vi "metadata_GetAttributes.vi"(0 "reference in":refnum<class "metadata.lvclass">, 1 "return data? (T)":bool=TRUE, 5 "error in (no error)":errorcluster) -> (14 "reference out":refnum<class "metadata.lvclass">, 15 "attributes ref":T13, 16 "attributes":T1={"MyAttribute"=0.0, "System Control"={"FPGA SW version"="", "TDMS file version"="", "Instrument"="", "Instrument model"="", "Instrument scanner"="", "Instrument clockrate (Mhz)"="", "Instrument tick time (us)"=""}, "file info"={"Time Stamp"=timestamp(0 s since 1904-01-01), "Filename"="", "Filepath"=path "", "User"="", "Experiment_name"="", "Curve_id"="", "number_segments"=0, "number_consecutive_scans"=0}, "Sample info"={"Sample name"="", "Sample species"=""}, "Cantilever info"={"spring constant calib method"="", "invOLS calib method"="", "thermal calib deflection channel"="", "model"="", "shape"="", "tip geometry"="", "Laser sum (V)"=0.0, "Laser power (mA)"=0.0, "invOLS_(nm/V)"=0.0, "spring constant nominal (N/m)"=0.0, "spring constant calib (N/m)"=0.0, "resosnance frequency air calib (Hz)"=0.0, "resosnance frequency calib (Hz)"=0.0, "quality factor"=0.0, "Acoefficident_GCI_(nN.s^1.3/m)"=0.0, "half angle (deg)"=0.0, "tip radius (m)"=0.0, "tip height (m)"=0.0, "system mount angle (deg)"=0.0}, "XYZ piezos"={"X stage piezo sensitivity (nm/V)"=0.0, "X stage piezo gain"=0.0, "X velocity (V/tick)"=0.0, "X closed loop"=FALSE, "Y stage piezo sensitivity (nm/V)"=0.0, "Y stage piezo gain"=0.0, "Y velocity (V/tick)"=0.0, "Y closed loop"=FALSE, "Z stage piezo sensitivity (nm/V)"=0.0, "Z stage piezo gain"=0.0, "Z closed loop"=FALSE, "X position (V)"=0.0, "Y position (V)"=0.0}, "Mapping"={"Mapping"=FALSE, "index"=0, "position row"=0, "position column"=0, "next position row"=0, "next position column"=0, "X initial position (V)"=0.0, "Y initial position (V)"=0.0, "X step size (V)"=0.0, "Y step size (V)"=0.0}, "Fcurve segment"=[], "Fast fpga segment"={"Fast start time trigger"=timestamp(0 s since 1904-01-01), "nb_points"=0, "sampling_rate_(S/s)"=0, "duration_(ticks)"=0}, "Chirp"={"f start (Hz)"=0.0, "f end (Hz)"=0.0, "Sweep type"=""}, "precision (6)"=6, "width (-)"=0, "Metadata"={"Property Names"=[], "Property Values"=[]}, "config filepath"=path "", "Section names []"=[], "Property names []"=[], "nb elements"=0}, 19 "error out":errorcluster)   [LabVIEW 2019, in "metadata.lvclass"]
doc: "Returns a reference and if wanted the actual data values of the attributes. This method is used by the subclasses to access parent attributes."
uses:
  metadata.lvclass
  C:/Program Files/National Instruments/LabVIEW 2019/vi.lib/addons/_AddQ/G#Object/G#Object.lvclass
  ObjectAttributesRef.ctl
  protected/ObjectAttributes.ctl
  System control parameters.ctl
  File info parameters.ctl
  Sample info parameters.ctl
  Cantilever info parameters.ctl
  XYZ piezos parameters.ctl
  Mapping parameters.ctl
  Fcurve segment.ctl
  Segment type--combobox.ctl
  fast fpga segment parameters.ctl
  Chirp added parameters.ctl
  Metadata output --cluster.ctl
  metadata.lvclass/metadata.ctl
  <vilib>/addons/_AddQ/G#Object/G#Object.lvclass
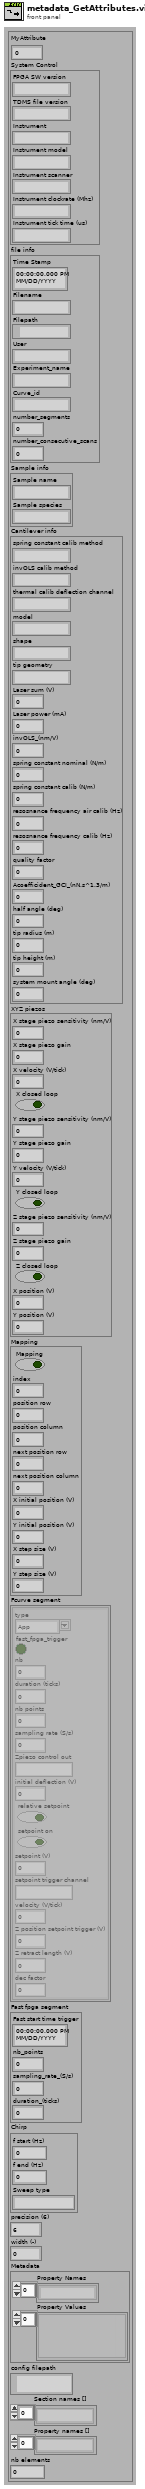
[diagram p1: front panel]
types:
  T1 = typedef "metadata.lvclass/ObjectAttributes.ctl" = cluster{"MyAttribute":dbl, "System Control":T2, "file info":T3, "Sample info":T4, "Cantilever info":T5, "XYZ piezos":T6, "Mapping":T7, "Fcurve segment":T8[], "Fast fpga segment":T10, "Chirp":T11, "precision (6)":i16, "width (-)":i16, "Metadata":T12, "config filepath":path, "Section names []":string[], "Property names []":string[], "nb elements":u16}
  T2 = typedef "metadata.lvclass/System control parameters.ctl" = cluster{"FPGA SW version":string, "TDMS file version":string, "Instrument":string, "Instrument model":string, "Instrument scanner":string, "Instrument clockrate (Mhz)":string, "Instrument tick time (us)":string}
  T3 = typedef "metadata.lvclass/File info parameters.ctl" = cluster{"Time Stamp":timestamp, "Filename":string, "Filepath":path, "User":string, "Experiment_name":string, "Curve_id":string, "number_segments":u8, "number_consecutive_scans":u32}
  T4 = typedef "metadata.lvclass/Sample info parameters.ctl" = cluster{"Sample name":string, "Sample species":string}
  T5 = typedef "metadata.lvclass/Cantilever info parameters.ctl" = cluster{"spring constant calib method":string, "invOLS calib method":string, "thermal calib deflection channel":string, "model":string, "shape":string, "tip geometry":string, "Laser sum (V)":dbl, "Laser power (mA)":dbl, "invOLS_(nm/V)":dbl, "spring constant nominal (N/m)":dbl, "spring constant calib (N/m)":dbl, "resosnance frequency air calib (Hz)":dbl, "resosnance frequency calib (Hz)":dbl, "quality factor":dbl, "Acoefficident_GCI_(nN.s^1.3/m)":dbl, "half angle (deg)":dbl, "tip radius (m)":dbl, "tip height (m)":dbl, "system mount angle (deg)":dbl}
  T6 = typedef "metadata.lvclass/XYZ piezos parameters.ctl" = cluster{"X stage piezo sensitivity (nm/V)":dbl, "X stage piezo gain":dbl, "X velocity (V/tick)":dbl, "X closed loop":bool, "Y stage piezo sensitivity (nm/V)":dbl, "Y stage piezo gain":dbl, "Y velocity (V/tick)":dbl, "Y closed loop":bool, "Z stage piezo sensitivity (nm/V)":dbl, "Z stage piezo gain":dbl, "Z closed loop":bool, "X position (V)":dbl, "Y position (V)":dbl}
  T7 = typedef "metadata.lvclass/Mapping parameters.ctl" = cluster{"Mapping":bool, "index":u16, "position row":u16, "position column":u16, "next position row":i16, "next position column":i16, "X initial position (V)":dbl, "Y initial position (V)":dbl, "X step size (V)":dbl, "Y step size (V)":dbl}
  T8 = typedef "metadata.lvclass/Fcurve segment.ctl" = cluster{"type":T9, "fast_fpga_trigger":bool, "nb":u8, "duration (ticks)":i64, "nb points":i32, "sampling rate (S/s)":u32, "Zpiezo control out":string, "initial deflection (V)":dbl, "relative setpoint":bool, "setpoint on":bool, "setpoint (V)":dbl, "setpoint trigger channel":string, "velocity (V/tick)":dbl, "Z position setpoint trigger (V)":dbl, "Z retract length (V)":dbl, "dec factor":u32}
  T9 = typedef "metadata.lvclass/Segment type--combobox.ctl" = string
  T10 = typedef "metadata.lvclass/fast fpga segment parameters.ctl" = cluster{"Fast start time trigger":timestamp, "nb_points":u32, "sampling_rate_(S/s)":u32, "duration_(ticks)":u32}
  T11 = typedef "metadata.lvclass/Chirp added parameters.ctl" = cluster{"f start (Hz)":dbl, "f end (Hz)":dbl, "Sweep type":string}
  T12 = typedef "metadata.lvclass/Metadata output --cluster.ctl" = cluster{"Property Names":string[], "Property Values":variant[]}
  T13 = typedef "metadata.lvclass/ObjectAttributesRef.ctl" = refnum<data-value>
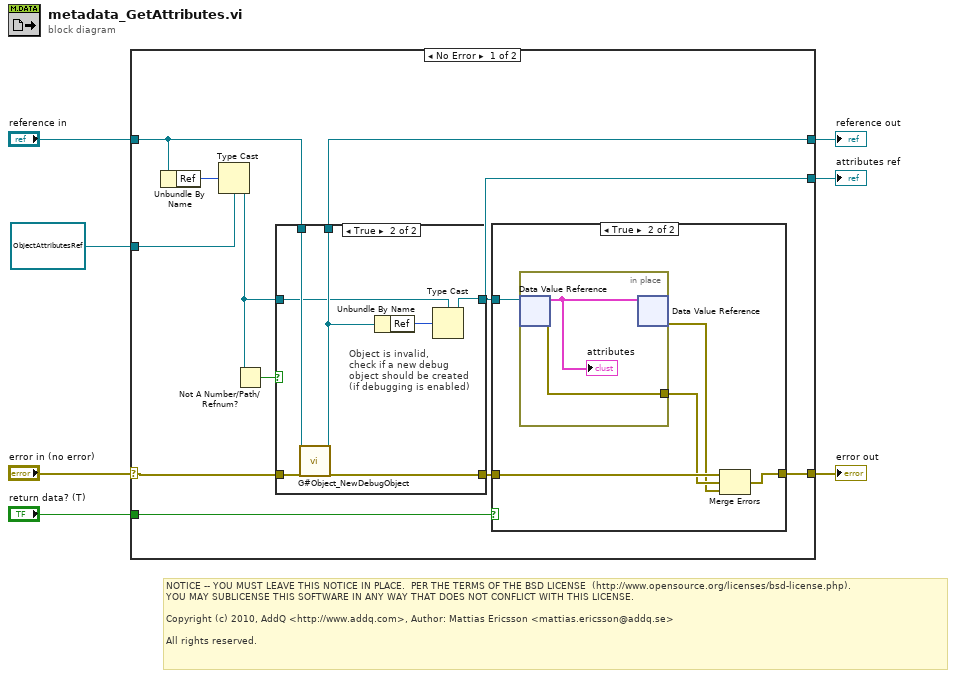
[diagram p0: block diagram]
diagram:
  # "NOTICE -- YOU MUST LEAVE THIS NOTICE IN PLACE.  PER THE TERMS OF THE BSD LICENSE  (http://www.opensource.org/licenses/bsd-license.php).\nYOU MAY SUBLICENSE THIS SOFTWARE IN ANY WAY THAT DOES NOT CONFLICT WITH THIS LICENSE.\n\nCopyright (c) 2010, AddQ <http://www.addq.com>, Author: Mattias Ericsson <mattias.ericsson@addq.se>\n\nAll rights reserved."
  n1 = case shown="No Error" "error in (no error)" {
    selector: "error in (no error)" -> [w14 w39]
    tunnel: [w17 w39] -> w6
    tunnel: [w11 w38] -> w4
    tunnel: "reference in" -> [w12 w38]
    tunnel: [w8 w37] -> w3
    tunnel: "return data? (T)" -> [w18 _]
    tunnel: T13 refnum ("attributes ref") -> [w10 w37]
    frame No Error {
      n2 = Unbundle By Name(w12) -> ("Ref"=w16:u32)
      n3 = Type Cast(type=w10, x=w16) -> (*(type *) &x=w9:T13)
      n4 = Not A Number/Path/Refnum?(number/path/refnum=w9) -> (NaN/Path/Refnum?=w13:bool)
      n5 = case shown="True" w13 {
        tunnel: [w21 w28] -> w15
        tunnel: w14 -> [w21 w27]
        tunnel: w12 -> [w20 w26]
        tunnel: [w20 w24] -> w11
        tunnel: w9 -> [w19 w23]
        tunnel: [w19 w22] -> w8
        frame False {
        }
        frame True {
          # "Object is invalid,\ncheck if a new debug\nobject should be created\n(if debugging is enabled)"
          n6 = call <vilib>:"G#Object_NewDebugObject.vi"("reference in"=w26, "error in (no error)"=w27) -> ("reference out"=w24:refnum<class "metadata.lvclass">, "error out"=w28:errorcluster)  [unwired: 16 in]
          n7 = Unbundle By Name(w24) -> ("Ref"=w25:u32)
          n8 = Type Cast(type=w23, x=w25) -> (*(type *) &x=w22:T13)
        }
      }
      n9 = case shown="True" w18 {
        tunnel: w8 -> [_ w34]
        tunnel: w15 -> [w29 w33]
        tunnel: [w29 w32] -> w17
        frame False {
        }
        frame True {
          n10 = in-place {
            in-place-border: [w36] -> w31
            n11 = in-place-dvr #1(w34) -> (w35:T1, w36:errorcluster)
            "attributes" <- w35
            n12 = in-place-dvr #1(w35) -> (w30:errorcluster)  [unwired: 1 out]
          }
          n13 = Merge Errors(w33, w31, w30) -> (w32:errorcluster)
        }
      }
    }
    frame Error {
    }
  }
  "error out" <- w6
  "reference out" <- w4
  "attributes ref" <- w3
